vi "Status to Glyph.vi"(11 "Status":T1=enum."Passed") -> (3 "Listbox Symbol Ring Constant":i32)   [LabVIEW 2020, in "LUnit Utilities.lvlib"]
uses:
  LUnit Utilities.lvlib
  Result/Status.ctl
  Result/Result.lvlib
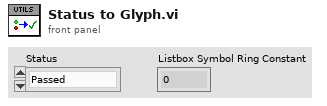
[diagram p1: front panel]
types:
  T1 = typedef "Result.lvlib/Status.ctl" = enum16{"", "Passed", "Failed", "Error", "Skipped", "Setup Error", "Broken", "Teardown Error"}
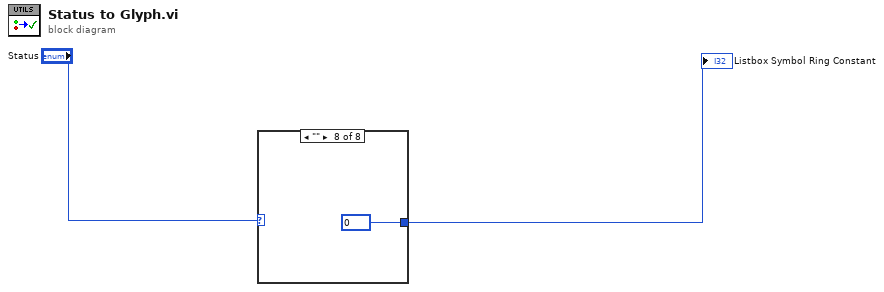
[diagram p0: block diagram]
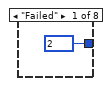
[diagram p2: hidden frame]
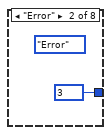
[diagram p3: hidden frame]
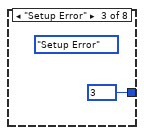
[diagram p4: hidden frame]
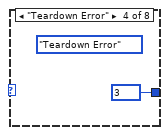
[diagram p5: hidden frame]
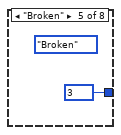
[diagram p6: hidden frame]
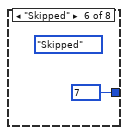
[diagram p7: hidden frame]
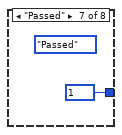
[diagram p8: hidden frame]
diagram:
  n1 = case shown="\"\"" "Status" {
    tunnel: [2 ("Listbox Symbol Ring Constant") 3 ("Listbox Symbol Ring Constant") 3 ("Listbox Symbol Ring Constant") 3 ("Listbox Symbol Ring Constant") 3 ("Listbox Symbol Ring Constant") 7 ("Listbox Symbol Ring Constant") 1 ("Listbox Symbol Ring Constant") 0 ("Listbox Symbol Ring Constant")] -> w2
    frame "Failed" {
    }
    frame "Error" {
      (unwired) Status."Error" ("Status")
    }
    frame "Setup Error" {
      (unwired) Status."Setup Error" ("Status")
    }
    frame "Teardown Error" {
      (unwired) Status."Teardown Error" ("Status")
    }
    frame "Broken" {
      (unwired) Status."Broken" ("Status")
    }
    frame "Skipped" {
      (unwired) Status."Skipped" ("Status")
    }
    frame "Passed" {
      (unwired) Status."Passed" ("Status")
    }
    frame "" {
    }
  }
  "Listbox Symbol Ring Constant" <- w2
